vi "Device Restart on Error.vi"() -> (1 "Restarted?":bool)   [LabVIEW 2017, in "Akwizycja.lvlib"]
uses:
  Akwizycja.lvlib
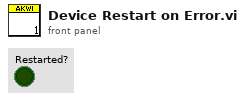
[diagram p1: front panel]
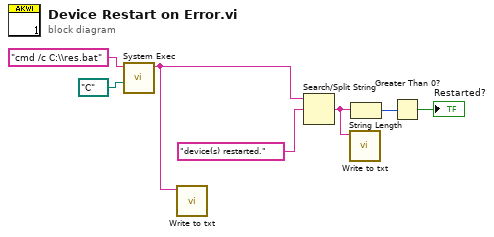
[diagram p0: block diagram]
diagram:
  n1 = call <vilib>:"System Exec.vi"("working directory"=path "C:/", "command line"="cmd /c C:\\res.bat") -> ("standard output"=w2:string)  [unwired: 6 in, 3 out]
  n2 = call "Write to txt.vi"("Input string"=w2) -> ()  [unwired: 10 in, 1 out]
  n3 = Search/Split String(string=w2, search string/char (-)="device(s) restarted." ("regular expression")) -> (match + rest of string=w1:string)  [unwired: 1 in, 2 out]
  n4 = call "Write to txt.vi"("Input string"=w1) -> ()  [unwired: 10 in, 1 out]
  n5 = String Length(string=w1) -> (length=w6:i32)
  n6 = Greater Than 0?(x=w6) -> (x > 0?=→"Restarted?":bool)
